vi "极限参数界面.vi"(8 "错误输入（无错误）":errorcluster, 10 "界面切换队列":refnum<queue>, 11 "VISA资源名称输入":refnum<visa-resource-name>) -> (0 "错误输出":errorcluster, 3 "VISA资源名称输出":refnum<visa-resource-name>)   [LabVIEW 2018]
panel:
  out "毫秒计时值":u32
  in  "枚举":T1(ring)
  in  "选项卡控件":enum32{"选项卡 1", "选项卡 2"}(tab)
  out "参数界面":bool
  out "读R906":bool
  out "读R905":bool
  out "读R904":bool
  out "写DDT32148+试用码3":dbl
  out "写DDT32146+试用码2":dbl
  out "写DDT32144+试用码1":dbl
  out "读DDT32160":dbl
  out "读DDT32162":dbl
  out "读DDT32164":dbl
  out "写R505+读R505":bool
  out "写R504+读R504":bool
  out "写R503+读R503":bool
  out "写R502+读R502":bool
  out "写DDT32586+Z2轴正限位":dbl
  out "写DDT32584+Z1轴正限位":dbl
  out "写DDT32582+Y轴正限位":dbl
  out "写DDT32580+X轴正限位":dbl
  out "DDT90356":dbl
  out "DDT90348":dbl
  out "自动界面":bool
  out "手动界面":bool
  out "参数界面":bool
  out "IO界面":bool
  out "产品界面":bool
  out "字符串":string
  out "DDT90352":dbl
  out "DDT90360":dbl
  out "通讯周期":dbl
  out "DT1184":T2(ring)
  # "X"
  # "Z1"
  # "Z2"
  # "Y"
  # "轴极限参数"
  # "X轴正极限位"
  # "Z1轴正极限位"
  # "Y轴正极限位"
  # "Z2轴正极限位"
  # "授权控制"
  # "已运行时间："
  # "试用码1："
  # "试用码1："
  # "试用码1："
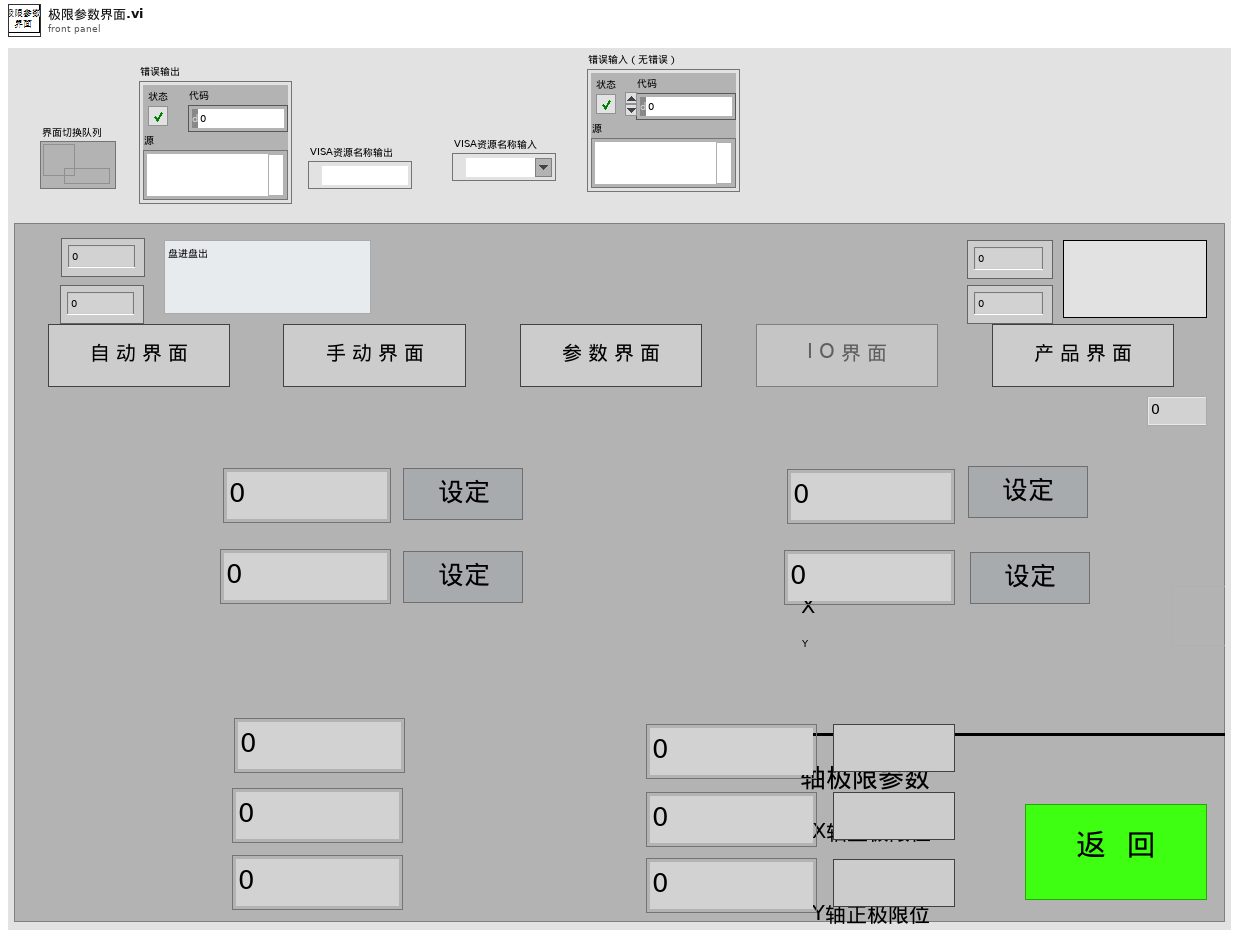
[diagram p1: front panel]
types:
  T1 = enum16{"读初始化", "读R504+8", "读R904+8", "读DDT32144+5", "读DDT32580+5", "读DDT32162+5", "读DDT90356", "读DT1184", "读DDT90348", ""}
  T2 = enum16{"盘进盘出", "卷进卷出", "盘进卷出", "管进盘出", "管进卷出", "卷进盘出", ""}
  T3 = enum8{"Enabled", "Disabled", "Disabled and Grayed Out"}
  T4 = typedef "数据簇.ctl" = cluster{"字符串":string, "数值":i32, "布尔":bool}
  T5 = typedef "lveventtype.ctl" = enum32{"Null", "Timeout", "Annotation Menu Selection", "Annotation Menu Selection?", "App Instance Close", "App Instance Close?", "Autoscale Range Change", "Bookmark Info Change", "Cell Edit", "Cell Edit?", "Cursor Grab", "Cursor Grab?", "Cursor Menu Selection", "Cursor Menu Selection?", "Cursor Move", "Cursor Release", "Data Change", "Direction Change", "Display State Change", "Drag Ended", "Drag Enter", "Drag Leave", "Drag Over", "Drag Source Update", "Drag Starting", "Drag Starting?", "Drop", "Exec State Change", "Key Down", "Key Down?", "Key Repeat", "Key Repeat?", "Key Up", "Listbox Double Click", "Menu Activation?", "Menu Selection (App)", "Menu Selection? (App)", "Menu Selection (User)", "Mouse Down", "Mouse Down?", "Mouse Enter", "Mouse Leave", "Mouse Move", "Mouse Up", "Mouse Wheel", "NI Security User Change (App)", "Pane Size", "Panel Close", "Panel Close?", "Panel Resize", "Plot Attribute Change", "Scale Range Change", "Shortcut Menu Activation?", "Shortcut Menu Selection (App)", "Shortcut Menu Selection? (App)", "Shortcut Menu Selection (User)", "Tree Double Click", "Tree Drag", "Tree Drag?", "Tree Drop", "Tree Drop?", "Tree Item Close", "Tree Item Close?", "Tree Item Open", "Tree Item Open?", "User Event", "Value Change"}
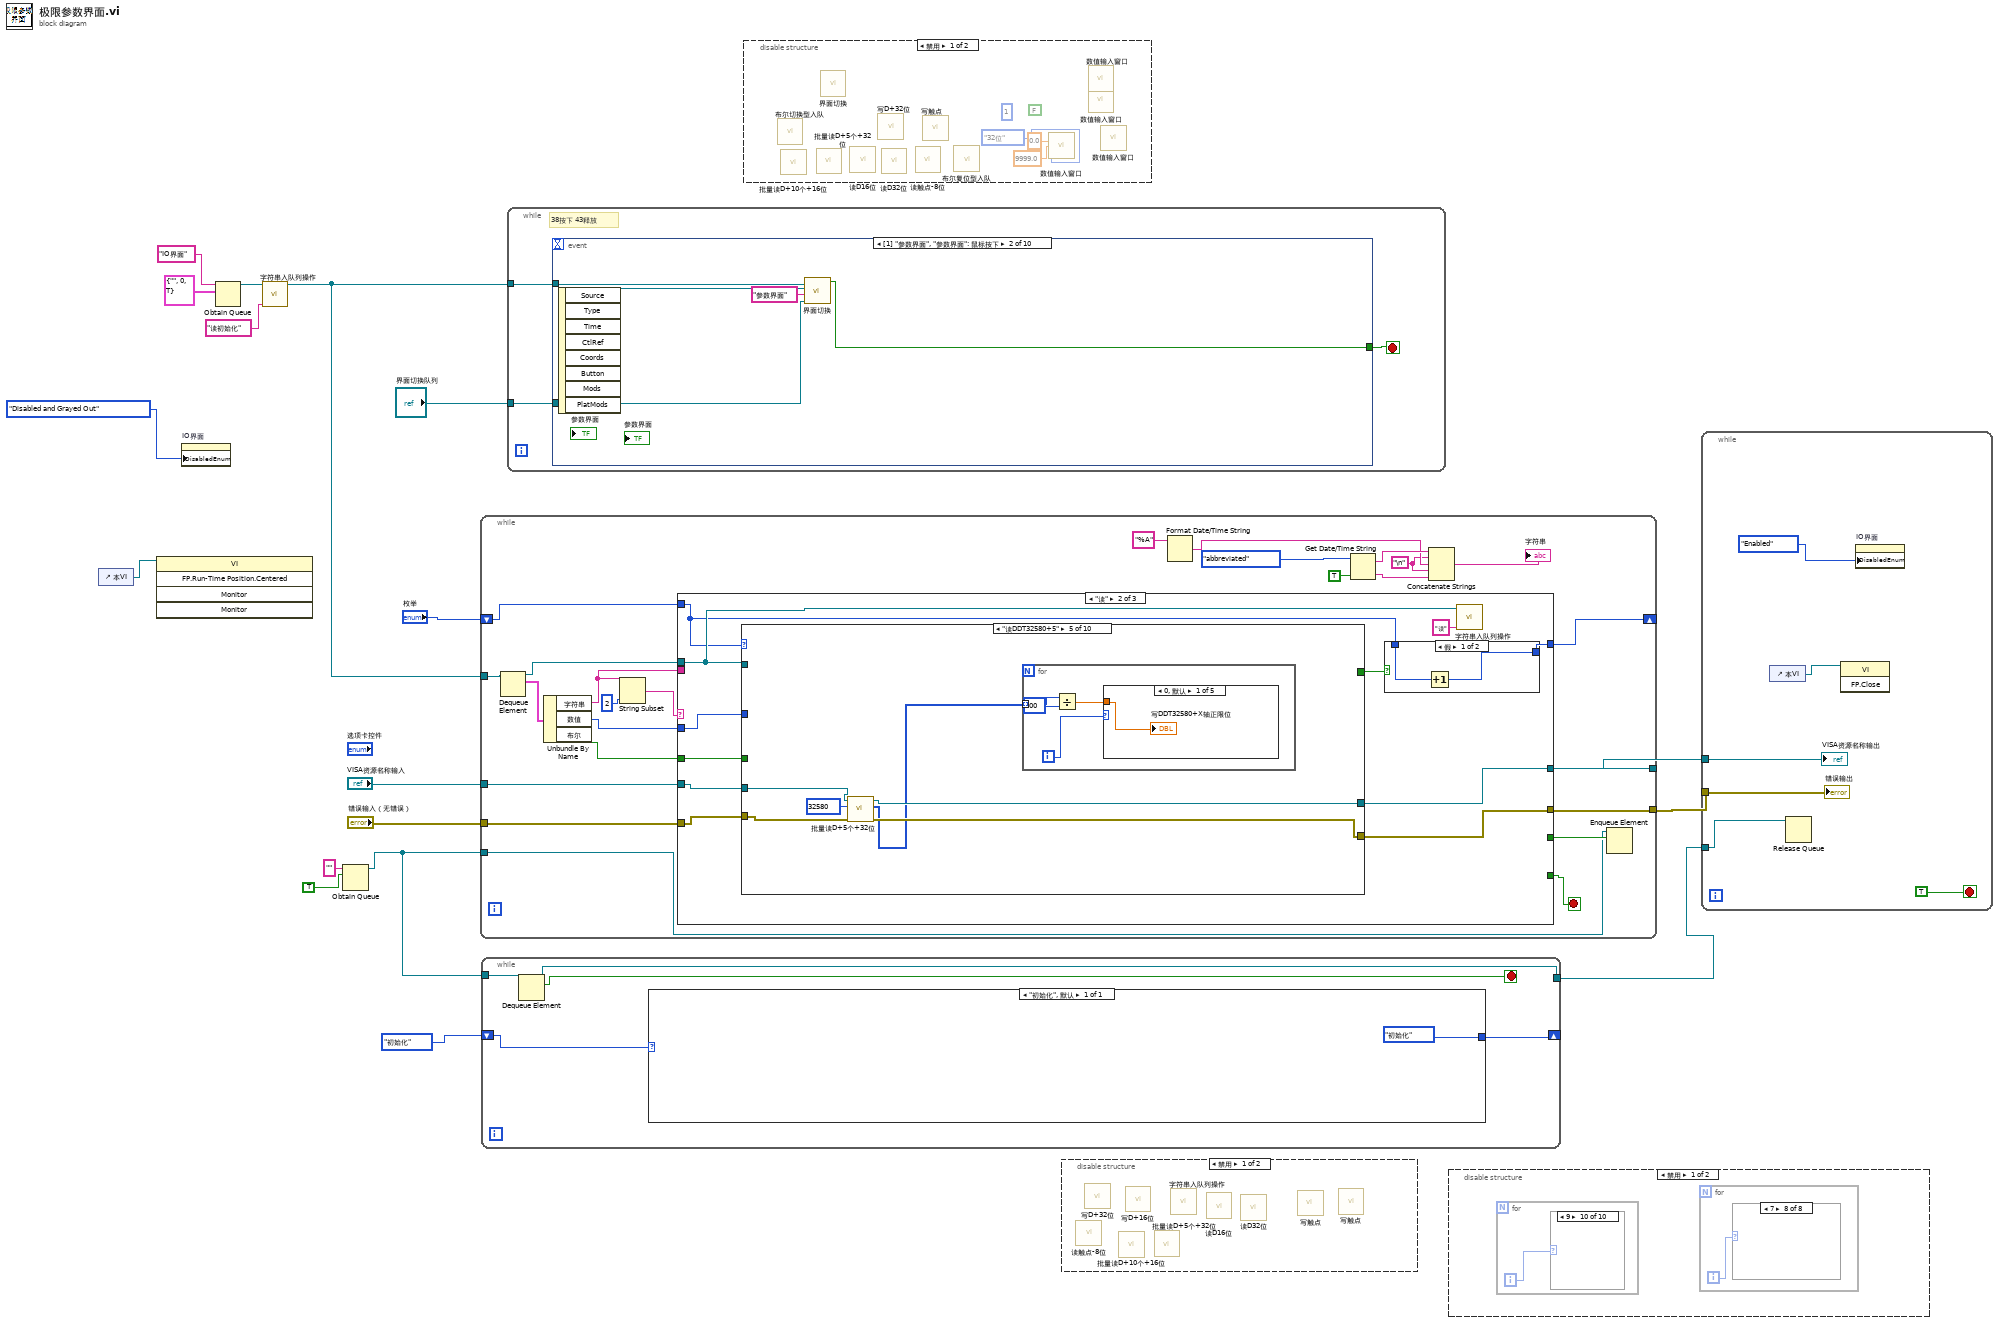
[diagram p0: block diagram]
diagram:
  n1 = control-ref of="本VI"() -> (w1:refnum<vi>)
  n2 = invoke class="VI" method="FP.Run-Time Position.Centered"(reference=w1) -> ()  [unwired: 4 in, 5 out]
  n3 = property on="IO界面" class="Bool"("DisabledEnum"=T3."Disabled and Grayed Out" ("禁用")) -> ()  [unwired: 2 in, 2 out]
  n4 = Obtain Queue(name (unnamed)="IO界面" ("名称（未命名）"), element data type=T4 {"字符串"="", "数值"=0, "布尔"=TRUE}) -> (queue out=w11:refnum<queue>)  [unwired: 3 in, 2 out]
  n5 = call "字符串入队列操作.vi"("字符消息入队列"="读初始化", "界面切换队列"=w11) -> ("队列输出"=w3:refnum<queue>)  [unwired: 9 in]
  n6 = Obtain Queue(name (unnamed)="" ("名称（未命名）"), element data type=TRUE) -> (queue out=w6:refnum<queue>)  [unwired: 3 in, 2 out]
  n7 = while {
    tunnel: w3 -> [w39]
    tunnel: "VISA资源名称输入" -> [w32]
    tunnel: "错误输入（无错误）" -> [w31]
    tunnel: [w30] -> w13
    tunnel: [w29] -> w12
    shift-right: [w26] -> _
    shift-left: "枚举" -> [w27]
    tunnel: w6 -> [w19]
    stop <- w21 stop-if-true
    w23 = "\n"
    n8 = Dequeue Element(queue=w39) -> (queue out=w36:refnum<queue>, element=w38:T4)  [unwired: 2 in, 2 out]
    n9 = Unbundle By Name(w38) -> ("字符串"=w33:string, "数值"=w35:i32, "布尔"=w34:bool)
    n10 = String Subset(string=w33, length (rest)=2 ("长度（剩余）")) -> (substring=w37:string)  [unwired: 1 in]
    n11 = case shown="\"读\"" w37 {
      selector: w37 -> [w46 _ _]
      tunnel: w36 -> [_ w54 w184]
      tunnel: w35 -> [_ w61 w183]
      tunnel: w34 -> [_ w60 w182]
      tunnel: w33 -> [_ _ w176]
      tunnel: w32 -> [w45 w59 w181]
      tunnel: w31 -> [w44 w58 w180]
      tunnel: [w45 w57 w178] -> w30
      tunnel: [w44 w56 w177] -> w29
      tunnel: [_ _ w179] -> w21
      tunnel: w27 -> [_ w52 _]
      tunnel: [_ w51 _] -> w26
      tunnel: [_ _ w174] -> w20
      frame "", Default {
        n12 = Concatenate Strings("无对应消息分支**" ("消息"), w46, "**" ("字符串"), "读写状态机" ("字符串")) -> (w48:string)
        n13 = One Button Dialog(message=w48) -> ()  [unwired: 1 in, 1 out]
      }
      frame "读" {
        n14 = case shown="\"读DDT32580+5\"" w52 {
          tunnel: w54 -> [_ _ _ _ _ _ _ _ _ _]
          tunnel: w61 -> [_ _ _ _ _ _ _ _ _ _]
          tunnel: w59 -> [w66 w73 w86 w97 w108 w122 w139 w148 w161 w173]
          tunnel: w58 -> [w65 w72 w85 w96 w107 w121 w138 w147 w160 w172]
          tunnel: [w66 w71 w84 w94 w105 w119 w137 w146 w159 w173] -> w57
          tunnel: [w65 w70 w83 w93 w104 w118 w136 w145 w158 w172] -> w56
          tunnel: w60 -> [_ _ _ _ _ _ _ _ _ _]
          tunnel: [_ _ _ _ _ _ _ _ _ TRUE] -> w53
          frame "读初始化" {
            n15 = Tick Count (ms)() -> (millisecond timer value=→"毫秒计时值":u32)
          }
          frame "读R504+8" {
            n16 = call "读触点-8位.vi"("error out"=w72, "触点类型"="R", "读取起始地址"="504", "VISA resource name out"=w73) -> ("error IO"=w70:errorcluster, "读取布尔数组"=w69:bool[], "VISA resource name out 2"=w71:refnum<visa-resource-name>)  [unwired: 4 in, 1 out]
            n17 = for {
              tunnel: w69 -> [w74] mode=indexing
              i -> [w75]
              n18 = case shown="2" w75 {
                tunnel: w74 -> [w76 w77 w78 w79 _ _ _ _]
                frame 0, Default {
                  "写R504+读R504" <- w76
                }
                frame 1 {
                  "写R505+读R505" <- w77
                }
                frame 2 {
                  "写R502+读R502" <- w78
                }
                frame 3 {
                  "写R503+读R503" <- w79
                }
                frame 4 {
                }
                frame 5 {
                }
                frame 6 {
                }
                frame 7 {
                }
              }
            }
          }
          frame "读R904+8" {
            n19 = call "读触点-8位.vi"("error out"=w85, "触点类型"="R", "读取起始地址"="904", "VISA resource name out"=w86) -> ("error IO"=w83:errorcluster, "读取布尔数组"=w82:bool[], "VISA resource name out 2"=w84:refnum<visa-resource-name>)  [unwired: 4 in, 1 out]
            n20 = for {
              tunnel: w82 -> [w87] mode=indexing
              i -> [w88]
              n21 = case shown="2" w88 {
                tunnel: w87 -> [w89 w90 w91 _ _ _ _ _]
                frame 0, Default {
                  "读R904" <- w89
                }
                frame 1 {
                  "读R905" <- w90
                }
                frame 2 {
                  "读R906" <- w91
                }
                frame 3 {
                }
                frame 4 {
                }
                frame 5 {
                }
                frame 6 {
                }
                frame 7 {
                }
              }
            }
          }
          frame "读DDT32144+5" {
            n22 = call "批量读D+5个+32位.vi"("error out"=w96, "读取D地址"=32144, "VISA resource name out"=w97) -> ("error IO"=w93:errorcluster, "数组"=w92:i32[], "VISA resource name out 2"=w94:refnum<visa-resource-name>)  [unwired: 5 in, 1 out]
            n23 = for {
              tunnel: w92 -> [w98] mode=indexing
              i -> [w99]
              n24 = case shown="0, 默认" w99 {
                tunnel: w98 -> [w100 w101 w102 _ _]
                frame 0, Default {
                  "写DDT32144+试用码1" <- w100
                }
                frame 1 {
                  "写DDT32146+试用码2" <- w101
                }
                frame 2 {
                  "写DDT32148+试用码3" <- w102
                }
                frame 3 {
                }
                frame 4 {
                }
              }
            }
          }
          frame "读DDT32580+5" {
            n25 = call "批量读D+5个+32位.vi"("error out"=w107, "读取D地址"=32580, "VISA resource name out"=w108) -> ("error IO"=w104:errorcluster, "数组"=w103:i32[], "VISA resource name out 2"=w105:refnum<visa-resource-name>)  [unwired: 5 in, 1 out]
            n26 = for {
              tunnel: w103 -> [w111] mode=indexing
              i -> [w112]
              n27 = Divide(x=w111, y=100) -> (x/y=w109:dbl)
              n28 = case shown="0, 默认" w112 {
                tunnel: w109 -> [w113 w114 w115 w116 _]
                frame 0, Default {
                  "写DDT32580+X轴正限位" <- w113
                }
                frame 1 {
                  "写DDT32582+Y轴正限位" <- w114
                }
                frame 2 {
                  "写DDT32584+Z1轴正限位" <- w115
                }
                frame 3 {
                  "写DDT32586+Z2轴正限位" <- w116
                }
                frame 4 {
                }
              }
            }
          }
          frame "读DDT32162+5" {
            n29 = call "批量读D+5个+32位.vi"("error out"=w121, "读取D地址"=32162, "VISA resource name out"=w122) -> ("error IO"=w118:errorcluster, "数组"=w117:i32[], "VISA resource name out 2"=w119:refnum<visa-resource-name>)  [unwired: 5 in, 1 out]
            n30 = for {
              tunnel: w117 -> [w123] mode=indexing
              i -> [w124]
              n31 = case shown="2" w124 {
                tunnel: w123 -> [w125 w126 w127 _ _]
                frame 0, Default {
                  "读DDT32160" <- w125
                }
                frame 1 {
                  "读DDT32162" <- w126
                }
                frame 2 {
                  "读DDT32164" <- w127
                }
                frame 3 {
                }
                frame 4 {
                }
              }
            }
          }
          frame "读DDT90356" {
            n32 = call "批量读D+5个+32位.vi"("error out"=w138, "读取D地址"=90356, "VISA resource name out"=w139) -> ("error IO"=w136:errorcluster, "数组"=w142:i32[], "VISA resource name out 2"=w137:refnum<visa-resource-name>)  [unwired: 5 in, 1 out]
            n33 = Index Array(array=w142, index #1=0 ("索引"), index #2=2 ("索引")) -> (element #1=w135:i32, element #2=w134:i32)
            n34 = To Double Precision Float(number=w135) -> (double precision float=w133:dbl)
            n35 = To Double Precision Float(number=w134) -> (double precision float=w130:dbl)
            n36 = Divide(x=w133, y=100.0) -> (x/y=→"DDT90356":dbl)
            n37 = Divide(x=w130, y=100.0) -> (x/y=→"DDT90360":dbl)
          }
          frame "读DT1184" {
            n38 = call "读D16位.vi"("error out"=w147, "读取D地址"=1184, "VISA resource name out"=w148) -> ("error IO"=w145:errorcluster, "数值"=→"DT1184":u32, "VISA resource name out 2"=w146:refnum<visa-resource-name>)  [unwired: 5 in, 1 out]
          }
          frame "读DDT90348" {
            n39 = call "批量读D+5个+32位.vi"("error out"=w160, "读取D地址"=90348, "VISA resource name out"=w161) -> ("error IO"=w158:errorcluster, "数组"=w165:i32[], "VISA resource name out 2"=w159:refnum<visa-resource-name>)  [unwired: 5 in, 1 out]
            n40 = Index Array(array=w165, index #1=0 ("索引"), index #2=2 ("索引")) -> (element #1=w157:i32, element #2=w156:i32)
            n41 = To Double Precision Float(number=w156) -> (double precision float=w151:dbl)
            n42 = To Double Precision Float(number=w157) -> (double precision float=w155:dbl)
            n43 = Divide(x=w151, y=100.0) -> (x/y=→"DDT90352":dbl)
            n44 = Divide(x=w155, y=100.0) -> (x/y=→"DDT90348":dbl)
          }
          frame "" {
            n45 = local read "毫秒计时值"() -> (w169:u32)
            n46 = Tick Count (ms)() -> (millisecond timer value=w170:u32)
            n47 = Subtract(x=w170, y=w169) -> (x-y=w168:u32)
            n48 = Divide(x=w168, y=u32 1000) -> (x/y=→"通讯周期":dbl)
          }
        }
        n49 = case shown="假" w53 {
          tunnel: w52 -> [w63 _]
          tunnel: [w62 _] -> w51
          frame False {
            n50 = Increment(x=w63) -> (x+1=w62:T1)
          }
          frame True {
          }
        }
        n51 = call "字符串入队列操作.vi"("字符消息入队列"="读", "界面切换队列"=w54) -> ()  [unwired: 9 in, 1 out]
      }
      frame "写" {
        n52 = call "状态匹配.vi"("输入状态"=w176) -> ("输出状态"=w175:string)  [unwired: 10 in]
        n53 = case shown="\"写退出\"" w175 {
          selector: w175 -> [w187 _ _ _ _]
          tunnel: w184 -> [_ _ _ _ w227]
          tunnel: w183 -> [_ w193 w210 _ _]
          tunnel: w182 -> [_ _ _ w221 _]
          tunnel: w181 -> [w186 w203 w214 w226 w232]
          tunnel: w180 -> [w185 w202 w213 w225 w231]
          tunnel: [_ _ _ _ w230] -> w179
          tunnel: [w186 w201 w212 w224 w232] -> w178
          tunnel: [w185 w200 w211 w223 w231] -> w177
          tunnel: w176 -> [_ w192 w204 w215 _]
          tunnel: [_ _ _ _ w230] -> w174
          frame "", Default {
            n54 = Concatenate Strings("无对应消息分支**" ("消息"), w187, "**" ("字符串"), "写状态机" ("字符串")) -> (w191:string)
            n55 = One Button Dialog(message=w191) -> ()  [unwired: 1 in, 1 out]
          }
          frame "写DT" {
            n56 = String Length(string=w192) -> (length=w198:i32)
            n57 = Subtract(x=w198, y=4) -> (x-y=w196:i32)
            n58 = String Subset(string=w192, offset (0)=4 ("偏移量(0)"), length (rest)=w196) -> (substring=w195:string)
            n59 = Decimal String To Number(string=w195) -> (number=w194:i32)  [unwired: 2 in, 1 out]
            n60 = call "写D+16位.vi"("error out"=w202, "输入数值"=w193, "输入地址D"=w194, "VISA resource name out"=w203) -> ("error out 2"=w200:errorcluster, "VISA resource name out 2"=w201:refnum<visa-resource-name>)  [unwired: 3 in, 3 out]
          }
          frame "写DDT" {
            n61 = String Length(string=w204) -> (length=w208:i32)
            n62 = Subtract(x=w208, y=5) -> ()  [unwired: 1 out]
            n63 = String Subset(string=w204, offset (0)=5 ("偏移量(0)")) -> (substring=w205:string)  [unwired: 1 in]
            n64 = Decimal String To Number(string=w205) -> (number=w206:i32)  [unwired: 2 in, 1 out]
            n65 = call "写D+32位.vi"("error out"=w213, "输入数值"=w210, "输入地址D"=w206, "VISA resource name out"=w214) -> ("error out 2"=w211:errorcluster, "VISA resource name out 2"=w212:refnum<visa-resource-name>)  [unwired: 4 in, 2 out]
          }
          frame "写R" {
            n66 = String Length(string=w215) -> (length=w219:i32)
            n67 = Subtract(x=w219, y=3) -> (x-y=w217:i32)
            n68 = String Subset(string=w215, offset (0)=3 ("偏移量(0)"), length (rest)=w217) -> (substring=w216:string)
            n69 = call "写触点.vi"("布尔"=w221, "error out"=w225, "触点类型"="R", "写入起始地址"=w216, "VISA resource name out"=w226) -> ("error IO"=w223:errorcluster, "VISA resource name out 2"=w224:refnum<visa-resource-name>)  [unwired: 4 in, 1 out]
          }
          frame "写退出" {
            w230 = TRUE
            n70 = Flush Queue(queue=w227) -> (queue out=w228:refnum<queue>, error out=w229:errorcluster)  [unwired: 1 in, 1 out]
            n71 = Release Queue(queue=w228, error in (no error)=w229) -> ()  [unwired: 1 in, 3 out]
          }
        }
      }
    }
    n72 = Format Date/Time String(time format string (%c)="%A" ("时间格式字符串(%c)")) -> (date/time string=w24:string)  [unwired: 2 in]
    n73 = Get Date/Time String(date format (0)=enum16{"short", "long", "abbreviated"}."abbreviated" ("日期格式(0)"), want seconds? (F)=TRUE ("需要秒？(F)")) -> (date string=w41:string, time string=w22:string)  [unwired: 1 in]
    n74 = Concatenate Strings(w41, w23, w24, w23, w22) -> (→"字符串":string)
    n75 = Enqueue Element(queue=w19, element=w20) -> ()  [unwired: 2 in, 3 out]
  }
  n76 = while {
    shift-right: [w236] -> _
    shift-left: enum16{"初始化"}."初始化" -> [w237]
    tunnel: w6 -> [w235]
    tunnel: [w233] -> w5
    stop <- w234 stop-if-true
    n77 = Dequeue Element(queue=w235) -> (queue out=w233:refnum<queue>, element=w234:bool)  [unwired: 2 in, 2 out]
    n78 = case shown="\"初始化\", 默认" w237 {
      tunnel: [enum16{"初始化"}."初始化"] -> w236
      frame "初始化", Default {
      }
    }
  }
  n79 = while {
    tunnel: w3 -> [w240]
    tunnel: "界面切换队列" -> [w239]
    stop <- w241 stop-if-true
    # "38按下 43释放"
    n80 = event shown="[1] \"参数界面\", \"参数界面\": 鼠标按下" {
      selector: _ -> [_ _ _ _ _ _ _ _ _ _]
      dyn-events: _ -> [_ _ _ _ _ _ _ _ _ _]
      timeout: _ -> [_ _ _ _ _ _ _ _ _ _]
      tunnel: [w245 w247 w252 _ _ _ w301 w306 _ w313] -> w241
      tunnel: w240 -> [w246 w251 w256 w264 w271 w300 w305 w310 _ w312]
      tunnel: w239 -> [w244 w250 w255 _ _ _ w304 w309 _ w311]
      event "IO界面": Mouse Down {
        n81 = event-data() -> ("CtlRef"=w243:refnum<vi>)  [unwired: 1 in, 7 out]
        n82 = call "界面切换.vi"("界面切换队列输入"=w244, "切换界面名称输入"="IO界面", "Bool引用句柄"=w243, "状态转移输入"=w246) -> ("布尔"=w245:bool)  [unwired: 7 in]
      }
      event "参数界面", "参数界面": Mouse Down {
        n83 = event-data() -> ("CtlRef"=w249:refnum<vi>)  [unwired: 1 in, 7 out]
        n84 = call "界面切换.vi"("界面切换队列输入"=w250, "切换界面名称输入"="参数界面", "Bool引用句柄"=w249, "状态转移输入"=w251) -> ("布尔"=w247:bool)  [unwired: 7 in]
      }
      event "产品界面": Mouse Down {
        n85 = event-data() -> ("CtlRef"=w254:refnum<vi>)  [unwired: 1 in, 7 out]
        n86 = call "界面切换.vi"("界面切换队列输入"=w255, "切换界面名称输入"="产品界面", "Bool引用句柄"=w254, "状态转移输入"=w256) -> ("布尔"=w252:bool)  [unwired: 7 in]
      }
      event "写DDT32580+X轴正限位", "写DDT32582+Y轴正限位", "写DDT32584+Z1轴正限位", "写DDT32586+Z2轴正限位": Mouse Down {
        n87 = event-data() -> ("CtlRef"=w267:refnum<vi>)  [unwired: 1 in, 7 out]
        n88 = property class="DigNum (严格)"(reference=w267) -> (reference out=w263:refnum<vi>, "Label.Text"=w266:string)  [unwired: 1 in, 1 out]
        n89 = Match Pattern(string=w266, regular expression="+" ("正则表达式")) -> (before substring=w258:string, after substring=w257:string)  [unwired: 1 in, 2 out]
        n90 = call "数值输入窗口.vi"("消息入队"=w264, "字符串"=w257, "字符消息入队列"=w258, "输入下限"=0.0, "输入上限"=999999999.0, "转换比例"=u32 100, "数据类型"=enum16{"32位", "16位"}."32位", "控件引用"=w263) -> ()  [unwired: 5 in, 3 out]
      }
      event "写R502+读R502", "写R503+读R503", "写R504+读R504", "写R505+读R505": Mouse Down {
        n91 = event-data() -> ("Type"=w270:T5, "CtlRef"=w276:refnum<vi>)  [unwired: 1 in, 6 out]
        n92 = property class="Bool"(reference=w276) -> (reference out=w269:refnum<vi>, "Label.Text"=w275:string)  [unwired: 1 in, 1 out]
        n93 = Two Button Dialog(message="确定设定？" ("消息")) -> (T button?=w272:bool)  [unwired: 2 in]
        n94 = Match Pattern(string=w275, regular expression="+" ("正则表达式")) -> (before substring=w268:string)  [unwired: 1 in, 3 out]
        n95 = case shown="真" w272 {
          tunnel: w271 -> [_ w286]
          tunnel: w270 -> [_ w285]
          tunnel: w269 -> [_ w284]
          tunnel: w268 -> [_ w283]
          frame False {
          }
          frame True {
            n96 = call "布尔复位型入队.vi"("队列输入"=w286, "数值"=w285, "控件引用"=w284, "字符消息入队列"=w283) -> ("队列输出"=w282:refnum<queue>, "控件引用 2"=w281:refnum<vi>, "字符消息出队列"=w280:string)  [unwired: 2 in]
            n97 = flat-sequence {
              tunnel: w282 -> [w289]
              tunnel: w281 -> [w288]
              tunnel: w280 -> [w287]
              tunnel: [w289] -> w279
              tunnel: [w288] -> w278
              tunnel: [w287] -> w277
              frame #0 {
                n98 = Wait (ms)(milliseconds to wait=u32 20 ("等待时间（毫秒）")) -> ()  [unwired: 1 out]
              }
            }
            n99 = call "布尔复位型入队.vi"("队列输入"=w279, "控件引用"=w278, "字符消息入队列"=w277) -> ()  [unwired: 3 in, 3 out]
          }
        }
      }
      event "写DDT32144+试用码1", "写DDT32146+试用码2", "写DDT32148+试用码3": Mouse Down {
        n100 = event-data() -> ("CtlRef"=w299:refnum<vi>)  [unwired: 1 in, 7 out]
        n101 = property class="DigNum (严格)"(reference=w299) -> ("Label.Text"=w298:string)  [unwired: 1 in, 2 out]
        n102 = Match Pattern(string=w298, regular expression="+" ("正则表达式")) -> (before substring=w296:string, after substring=w295:string)  [unwired: 1 in, 2 out]
        n103 = call "数值输入窗口.vi"("消息入队"=w300, "字符串"=w295, "字符消息入队列"=w296, "输入下限"=0.0, "输入上限"=999999999.0, "转换比例"=u32 1, "数据类型"=enum16{"32位", "16位"}."32位") -> ()  [unwired: 6 in, 3 out]
      }
      event "手动界面": Mouse Down {
        n104 = event-data() -> ("CtlRef"=w303:refnum<vi>)  [unwired: 1 in, 7 out]
        n105 = call "界面切换.vi"("界面切换队列输入"=w304, "切换界面名称输入"="手动界面", "Bool引用句柄"=w303, "状态转移输入"=w305) -> ("布尔"=w301:bool)  [unwired: 7 in]
      }
      event "自动界面": Mouse Down {
        n106 = event-data() -> ("CtlRef"=w308:refnum<vi>)  [unwired: 1 in, 7 out]
        n107 = call "界面切换.vi"("界面切换队列输入"=w309, "切换界面名称输入"="自动界面", "Bool引用句柄"=w308, "状态转移输入"=w310) -> ("布尔"=w306:bool)  [unwired: 7 in]
      }
      event Timeout {
        n108 = event-data() -> ()  [unwired: 1 in, 3 out]
      }
      event Panel Close? {
        n109 = event-data() -> ()  [unwired: 1 in, 4 out]
        n110 = Two Button Dialog(message="确定退出程序？" ("消息")) -> (T button?=w314:bool)  [unwired: 2 in]
        n111 = case shown="真" w314 {
          tunnel: [_ TRUE] -> w313
          tunnel: w312 -> [_ w319]
          tunnel: w311 -> [_ w318]
          frame False {
          }
          frame True {
            n112 = call "字符串入队列操作.vi"("字符消息入队列"="退出", "界面切换队列"=w318) -> ()  [unwired: 9 in, 1 out]
            n113 = call "字符串入队列操作.vi"("字符消息入队列"="写退出", "界面切换队列"=w319) -> ()  [unwired: 9 in, 1 out]
          }
        }
        n114 = event-data("Discard?"=TRUE ("放弃？")) -> ()  [unwired: 1 in, 1 out]
      }
    }
  }
  n115 = disable-structure shown="禁用" {
    frame Disabled {
      (unwired) u32 1 ("转换比例")
      (unwired) FALSE ("忽略数值上下限")
      n116 = call "布尔切换型入队.vi"() -> ()  [unwired: 12 in]
      n117 = call "批量读D+10个+16位.vi"() -> ()  [unwired: 8 in, 4 out]
      n118 = call "批量读D+5个+32位.vi"() -> ()  [unwired: 8 in, 4 out]
      n119 = call "界面切换.vi"() -> ()  [unwired: 11 in, 1 out]
      n120 = call "读D16位.vi"() -> ()  [unwired: 8 in, 4 out]
      n121 = call "写D+32位.vi"() -> ()  [unwired: 8 in, 4 out]
      n122 = call "读D32位.vi"() -> ()  [unwired: 9 in, 3 out]
      n123 = call "读触点-8位.vi"() -> ()  [unwired: 8 in, 4 out]
      n124 = call "写触点.vi"() -> ()  [unwired: 9 in, 3 out]
      n125 = call "布尔复位型入队.vi"() -> ()  [unwired: 6 in, 3 out]
      n126 = call "数值输入窗口.vi"("输入下限"=0.0, "输入上限"=9999.0, "数据类型"=enum16{"32位", "16位"}."32位") -> ("转换比例"=w325:u32)  [unwired: 9 in, 3 out]
      n127 = call "数值输入窗口.vi"() -> ()  [unwired: 13 in, 3 out]
      n128 = call "数值输入窗口.vi"() -> ()  [unwired: 13 in, 3 out]
      n129 = call "数值输入窗口.vi"() -> ()  [unwired: 13 in, 3 out]
    }
    frame Enabled {
    }
  }
  n130 = disable-structure shown="禁用" {
    frame Disabled {
      n131 = call "读触点-8位.vi"() -> ()  [unwired: 8 in, 4 out]
      n132 = call "写D+32位.vi"() -> ()  [unwired: 8 in, 4 out]
      n133 = call "批量读D+10个+16位.vi"() -> ()  [unwired: 8 in, 4 out]
      n134 = call "写D+16位.vi"() -> ()  [unwired: 7 in, 5 out]
      n135 = call "批量读D+5个+32位.vi"() -> ()  [unwired: 8 in, 4 out]
      n136 = call "字符串入队列操作.vi"() -> ()  [unwired: 11 in, 1 out]
      n137 = call "读D16位.vi"() -> ()  [unwired: 8 in, 4 out]
      n138 = call "读D32位.vi"() -> ()  [unwired: 9 in, 3 out]
      n139 = call "写触点.vi"() -> ()  [unwired: 9 in, 3 out]
      n140 = call "写触点.vi"() -> ()  [unwired: 9 in, 3 out]
    }
    frame Enabled {
    }
  }
  n141 = disable-structure shown="禁用" {
    frame Disabled {
      n142 = for {
        i -> [w327]
        n143 = case shown="9" w327 {
          frame 0, Default {
          }
          frame 1 {
          }
          frame 2 {
          }
          frame 3 {
          }
          frame 4 {
          }
          frame 5 {
          }
          frame 6 {
          }
          frame 7 {
          }
          frame 8 {
          }
          frame 9 {
          }
        }
      }
      n144 = for {
        i -> [w326]
        n145 = case shown="7" w326 {
          frame 0, Default {
          }
          frame 1 {
          }
          frame 2 {
          }
          frame 3 {
          }
          frame 4 {
          }
          frame 5 {
          }
          frame 6 {
          }
          frame 7 {
          }
        }
      }
    }
    frame Enabled {
    }
  }
  n146 = while {
    tunnel: w13 -> [w331]
    tunnel: w12 -> [w330]
    tunnel: w5 -> [w329]
    stop <- TRUE stop-if-true
    n147 = control-ref of="本VI"() -> (w332:refnum<vi>)
    n148 = Release Queue(queue=w329) -> ()  [unwired: 2 in, 3 out]
    n149 = invoke class="VI" method="FP.Close"(reference=w332) -> ()  [unwired: 2 in, 3 out]
    n150 = property on="IO界面" class="Bool"("DisabledEnum"=T3."Enabled" ("禁用")) -> ()  [unwired: 2 in, 2 out]
    "VISA资源名称输出" <- w331
    "错误输出" <- w330
  }
